vi "TDMS_readTable.vi"() -> ()   [LabVIEW 2011]
panel:
  out "string":string[][](array[string])
  out "numeric":dbl[][](array[numeric])
  out "error out":errorcluster
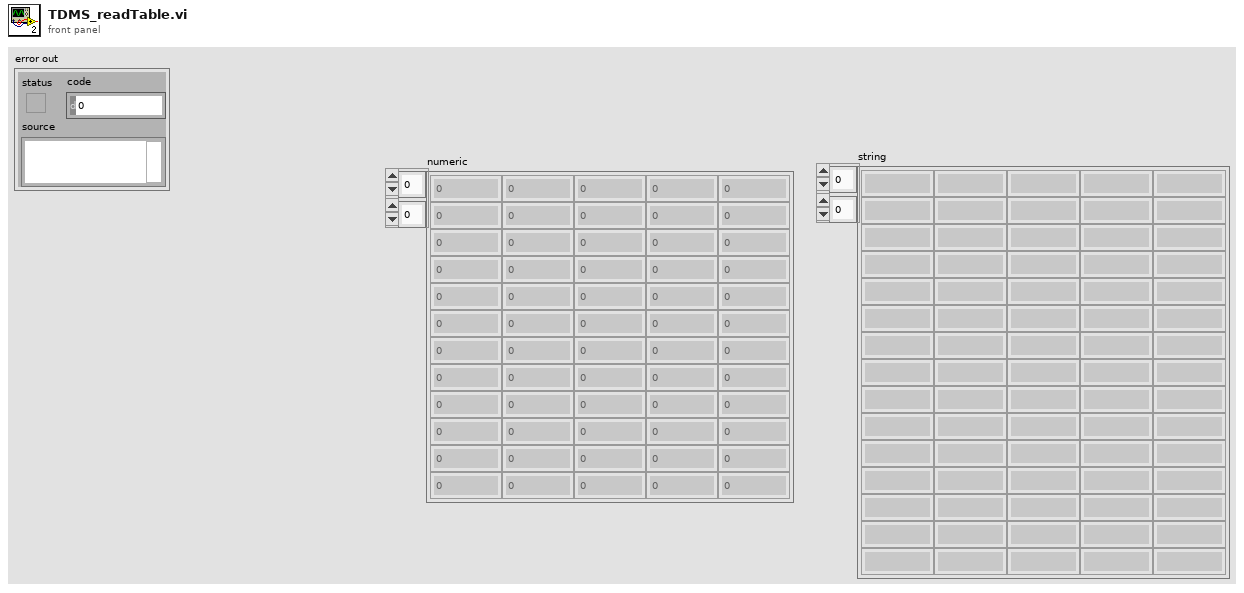
[diagram p1: front panel]
types:
  T1 = enum16{"open", "open or create", "create or replace", "create", "open (read-only)"}
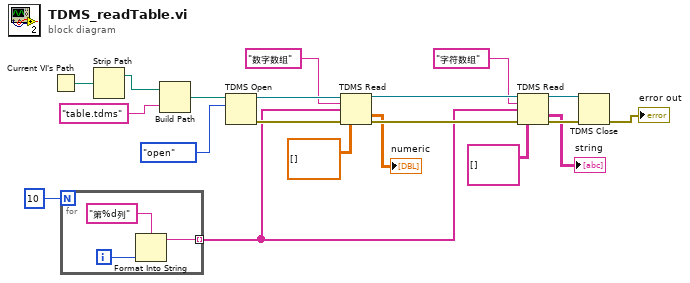
[diagram p0: block diagram]
diagram:
  n1 = Current VI's Path() -> (path=w20:path)
  n2 = for {
    N: 10 -> [_]
    tunnel: [w22] -> w4 mode=indexing
    i -> [w23]
    n3 = Format Into String(format string="第%d列" ("initial string"), w23) -> (resulting string=w22:string)  [unwired: 2 in, 1 out]
  }
  n4 = Strip Path(path=w20) -> (stripped path=w19:path)  [unwired: 1 out]
  n5 = Build Path(base path=w19, name or relative path="table.tdms") -> (appended path=w9:path)
  n6 = TDMS Open(10:T1."open" ("operation (0:open)"), 11:w9) -> (0:w8:errorcluster, 3:w17:refnum<k34>)  [unwired: 4 in]
  n7 = TDMS Read(0:w17, 5:"数字数组" ("group name in (Untitled)"), 7:w4, 11:w8, 12:dbl[][] []) -> (4:w16:refnum<k34>, 10:→"numeric":dbl[][], 15:w7:errorcluster)  [unwired: 3 in, 3 out]
  n8 = TDMS Read(0:w16, 5:"字符数组" ("group name in (Untitled)"), 7:w4, 11:w7, 12:string[][] [] ("channel name(s) in")) -> (4:w15:refnum<k34>, 10:→"string":string[][], 15:w14:errorcluster)  [unwired: 3 in, 3 out]
  n9 = TDMS Close(8:w14, 11:w15) -> (0:→"error out":errorcluster)  [unwired: 1 out]
